vi "rs3 get failed function.vi"(8 "error in (no error)":errorcluster, 11 "error in":u64) -> (0 "error out":errorcluster, 2 "error out":u64, 3 "Failed Function":string)   [LabVIEW 2019, in "libRealSense3.lvlib"]
doc: "const char * rs_get_failed_function (const rs_error * error);"
uses:
  libRealSense3.lvlib
  Intel RealSense SDK 2.0/bin/x86/realsense2.dll
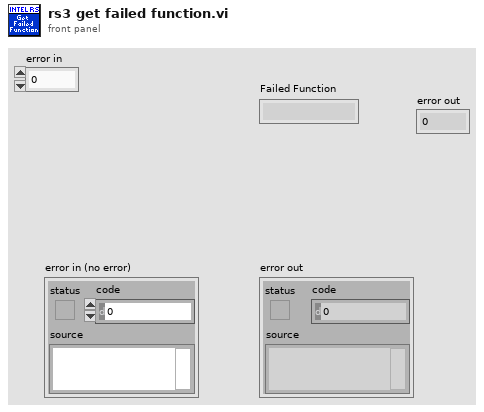
[diagram p1: front panel]
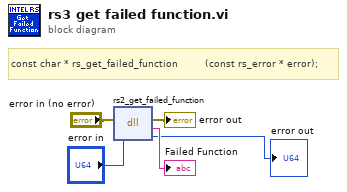
[diagram p0: block diagram]
diagram:
  # "const char * rs_get_failed_function         (const rs_error * error);"
  n1 = dll-call lib="C:/Program Files (x86)/Intel RealSense SDK 2.0/bin/x86/realsense2.dll" fn="rs2_get_failed_function"(error in="error in (no error)", "error"="error in") -> (error out=→"error out":errorcluster, "return type"=→"Failed Function":string, "error"=→"error out":u64)  [unwired: 2 in, 1 out]
